vi "PicoScope2000ExampleBlock.vi"() -> ()   [LabVIEW 2017]
uses:
  PS2000.dll
panel:
  out "Handle in":i16
  out "handle out":i16
  in  "Sweeps":u32
  in  "Sweep Type":enum16{"Up", "Down", "Up/Down", "Down/Up"}(ring)
  in  "Dwell Time":sgl
  in  "Increment":sgl
  in  "Stop Frequency":sgl=1000.0
  in  "Start Frequency":sgl=1000.0
  in  "Waveform Type":T1(ring)
  in  "Peak to Peak":u32=1000000
  in  "Offset Voltage":i32
  in  "Source":i16(ring)=5 items=["Ch A", "Ch B", "Ch C", "Ch D", "Ext", "None"]
  in  "Voltage mV":i16=1400 min=0 max=20000 step=1
  out "Max number of samples you can use":i32=3967
  in  "Range":i16(ring)=8 items=["20V"=10, "10V"=9, "5V"=8, "2V"=7, "1V"=6, "500mV"=5, "200mV"=4, "100mV"=3, "50mV"=2]
  in  "Range":i16(ring)=8 items=["20V"=10, "10V"=9, "5V"=8, "2V"=7, "1V"=6, "500mV"=5, "200mV"=4, "100mV"=3, "50mV"=2]
  out "?":waveform(dbl)[](graph)=[{"t0"=timestamp(3612161019.70979 s since 1904-01-01), "dt"=8e-08, "Y"=array[1256 elements]}, {"t0"=timestamp(3612161019.70979 s since 1904-01-01), "dt"=8e-08, "Y"=array[1256 elements]}, {"t0"=timestamp(3612161019.70979 s since 1904-01-01), "dt"=8e-08, "Y"=array[1256 elements]}, {"t0"=timestamp(3612161019.70979 s since 1904-01-01), "dt"=8e-08, "Y"=array[1256 elements]}]
  in  "Enabled":bool=TRUE
  in  "Enabled":bool=TRUE
  in  "DC":i16(ring) items=["AC", "DC"]
  in  "DC":i16(ring)=1 items=["AC", "DC"]
  in  "No. of samples":i32=1256 min=0
  in  "Timebase":i16=3 min=0 max=14 step=1
  in  "Auto Trigger ms":i16 min=0 max=5000 step=100
  in  "Delay":i16 min=-100 max=100 step=1
  in  "Direction":i16(ring) items=["Rising", "Falling"]
  in  "stop":bool
  # "Trigger"
  # "Channel A"
  # "Channel B"
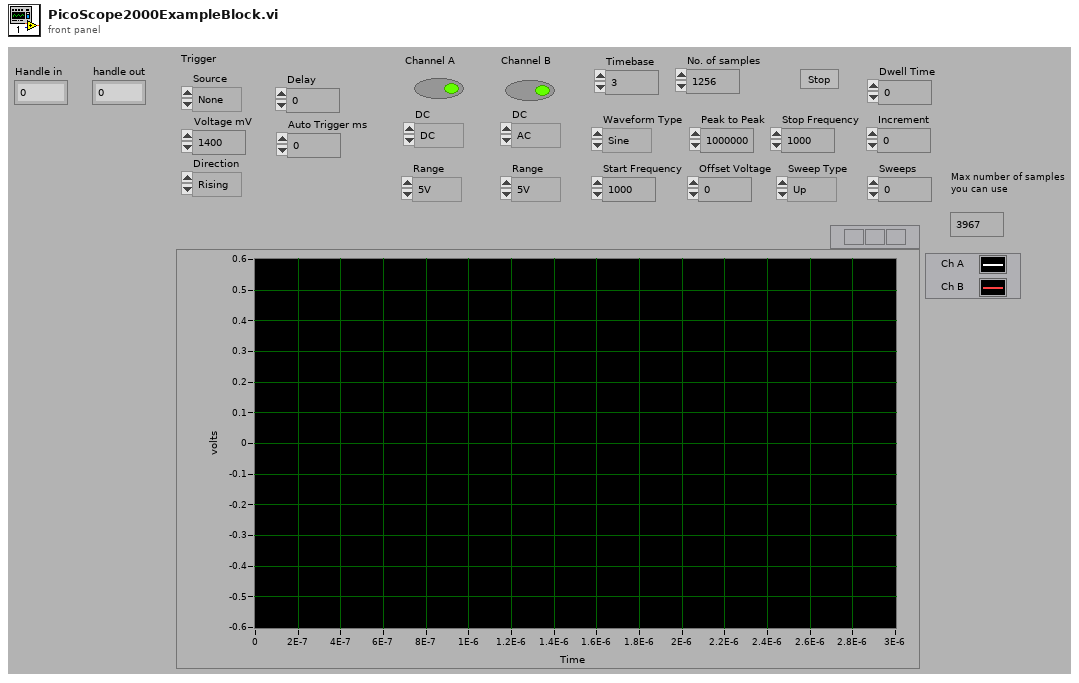
[diagram p1: front panel]
types:
  T1 = enum16{"Sine", "Square", "Triangle", "Rampup", "Rampdown"}
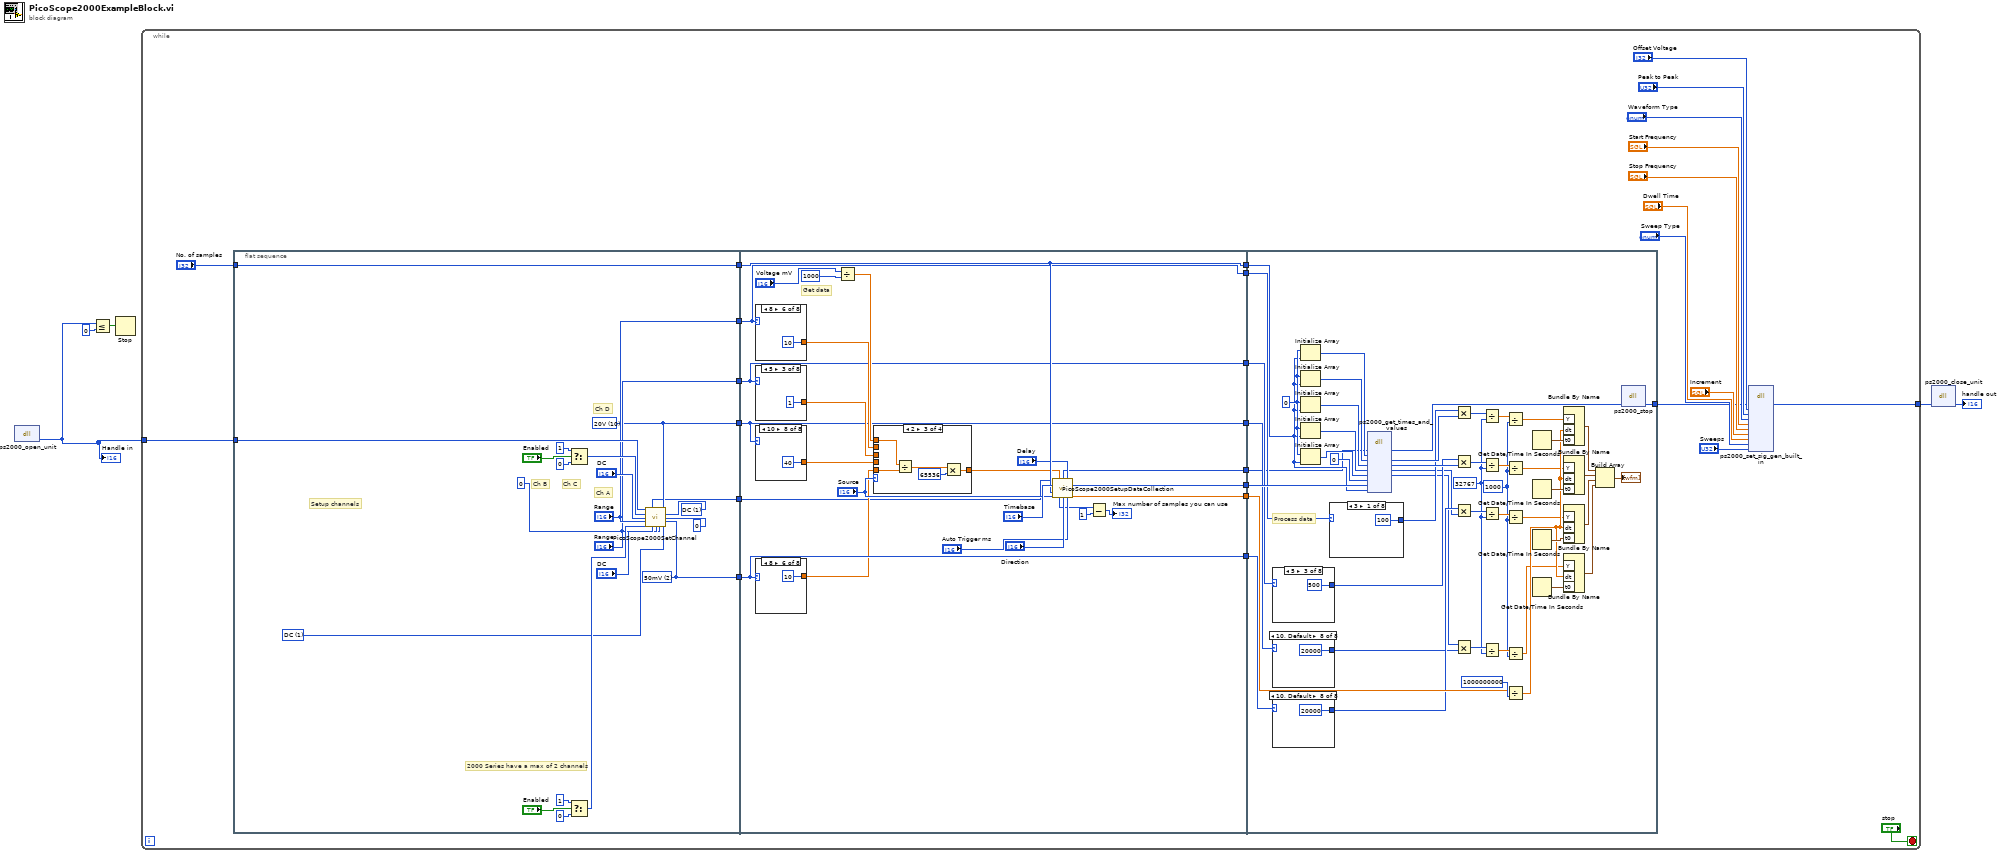
[diagram p0: block diagram]
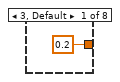
[diagram p2: hidden frame]
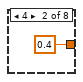
[diagram p3: hidden frame]
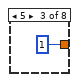
[diagram p4: hidden frame]
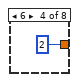
[diagram p5: hidden frame]
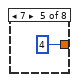
[diagram p6: hidden frame]
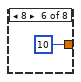
[diagram p7: hidden frame]
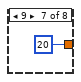
[diagram p8: hidden frame]
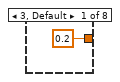
[diagram p9: hidden frame]
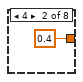
[diagram p10: hidden frame]
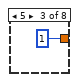
[diagram p11: hidden frame]
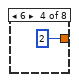
[diagram p12: hidden frame]
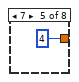
[diagram p13: hidden frame]
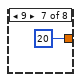
[diagram p14: hidden frame]
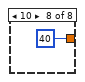
[diagram p15: hidden frame]
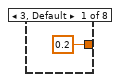
[diagram p16: hidden frame]
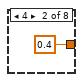
[diagram p17: hidden frame]
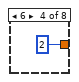
[diagram p18: hidden frame]
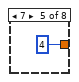
[diagram p19: hidden frame]
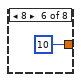
[diagram p20: hidden frame]
diagram:
  n1 = dll-call lib="PS2000.dll" fn="ps2000_open_unit" label="OpenUnit"() -> ("Handle"=w2:i16)  [unwired: 3 in, 2 out]
  "Handle in" <- w2
  n2 = Less Or Equal?(x=w2, y=i16 0) -> (x <= y?=w4:bool)
  n3 = Stop(stop? (T)=w4) -> ()
  n4 = while {
    tunnel: w2 -> [w32]
    tunnel: [w20] -> w5
    stop <- "stop" stop-if-true
    n5 = flat-sequence {
      tunnel: w32 -> [w48]
      tunnel: "No. of samples" -> [w34]
      tunnel: [w34] -> w19
      tunnel: [w35] -> w18
      tunnel: ["Range"] -> w17
      tunnel: ["Range"] -> w16
      tunnel: [w39] -> w15
      tunnel: [w38] -> w14
      tunnel: w19 -> [w75]
      tunnel: [w55] -> w13
      tunnel: w18 -> [w56]
      tunnel: [w75] -> w12
      tunnel: [w76] -> w11
      tunnel: w17 -> [w62]
      tunnel: [w62] -> w10
      tunnel: w16 -> [w63]
      tunnel: [w63] -> w9
      tunnel: [w74] -> w8
      tunnel: w15 -> [w60]
      tunnel: [w60] -> w7
      tunnel: w14 -> [w59]
      tunnel: [w59] -> w6
      tunnel: [w132] -> w21
      tunnel: w13 -> [w133]
      tunnel: w12 -> [w137]
      tunnel: w11 -> [w177]
      tunnel: w10 -> [w164]
      tunnel: w9 -> [w165]
      tunnel: w8 -> [w162]
      tunnel: w7 -> [w151]
      tunnel: w6 -> [w150]
      frame #0 {
        w40 = i16 1 items=["AC", "DC"] ("DC")
        w38 = i16 10 items=["20V"=10, "10V"=9, "5V"=8, "2V"=7, "1V"=6, "500mV"=5, "200mV"=4, "100mV"=3, "50mV"=2] ("Range")
        w41 = i16 1 items=["AC", "DC"] ("DC")
        w39 = i16 2 items=["20V"=10, "10V"=9, "5V"=8, "2V"=7, "1V"=6, "500mV"=5, "200mV"=4, "100mV"=3, "50mV"=2] ("Range")
        # "2000 Series have a max of 2 channels"
        # "Ch C"
        # "Ch D"
        # "Ch B"
        # "Ch A"
        # "Setup channels"
        n6 = Select(t=1, s="Enabled", f=0) -> (s? t:f=w47:i32)
        n7 = Select(t=1, s="Enabled", f=0) -> (s? t:f=w44:i32)
        n8 = call "PicoScope2000SetChannel.vi"("Handle in"=w48, "Channel D range"=w38, "Channel A enabled"=w47, "Channel D dc"=w40, "Channel A dc"="DC", "Channel D enabled"=0, "Channel A range"="Range", "Channel C range"=w39, "Channel B enabled"=w44, "Channel B dc"="DC", "Channel B range"="Range", "Channel C enabled"=0, "Channel C dc"=w41) -> ("Handle out"=w35:i16)  [unwired: 2 in]
      }
      frame #1 {
        # "Get data"
        n9 = case shown="8" w62 {
          tunnel: [0.2 0.4 1 2 4 10 20 40] -> w66
          frame 3, Default {
          }
          frame 4 {
          }
          frame 5 {
          }
          frame 6 {
          }
          frame 7 {
          }
          frame 8 {
          }
          frame 9 {
          }
          frame 10 {
          }
        }
        n10 = case shown="5" w63 {
          tunnel: [0.2 0.4 1 2 4 10 20 40] -> w65
          frame 3, Default {
          }
          frame 4 {
          }
          frame 5 {
          }
          frame 6 {
          }
          frame 7 {
          }
          frame 8 {
          }
          frame 9 {
          }
          frame 10 {
          }
        }
        n11 = case shown="10" w59 {
          tunnel: [0.2 0.4 1 2 4 10 20 40] -> w57
          frame 3, Default {
          }
          frame 4 {
          }
          frame 5 {
          }
          frame 6 {
          }
          frame 7 {
          }
          frame 8 {
          }
          frame 9 {
          }
          frame 10 {
          }
        }
        n12 = case shown="8" w60 {
          tunnel: [0.2 0.4 1 2 4 10 20 40] -> w58
          frame 3, Default {
          }
          frame 4 {
          }
          frame 5 {
          }
          frame 6 {
          }
          frame 7 {
          }
          frame 8 {
          }
          frame 9 {
          }
          frame 10 {
          }
        }
        n13 = Divide(x="Voltage mV", y=1000) -> (x/y=w67:dbl)
        n14 = case shown="2" "Source" {
          tunnel: w66 -> [w115 _ _ _]
          tunnel: w65 -> [_ w117 _ _]
          tunnel: w67 -> [w116 w118 w123 w128]
          tunnel: [w112 w119 w124 w129] -> w61
          tunnel: w58 -> [_ _ w122 _]
          tunnel: w57 -> [_ _ _ w127]
          frame 0, Default {
            n15 = Divide(x=w116, y=w115) -> (x/y=w114:dbl)
            n16 = Multiply(x=w114, y=65536) -> (x*y=w112:dbl)
          }
          frame 1 {
            n17 = Divide(x=w118, y=w117) -> (x/y=w121:dbl)
            n18 = Multiply(x=w121, y=65536) -> (x*y=w119:dbl)
          }
          frame 2 {
            n19 = Divide(x=w123, y=w122) -> (x/y=w126:dbl)
            n20 = Multiply(x=w126, y=65536) -> (x*y=w124:dbl)
          }
          frame 3 {
            n21 = Divide(x=w128, y=w127) -> (x/y=w131:dbl)
            n22 = Multiply(x=w131, y=65536) -> (x*y=w129:dbl)
          }
        }
        n23 = call "PicoScope2000SetupDataCollection.vi"("Handle in"=w56, "Threshold"=w61, "Delay"="Delay", "Timebase"="Timebase", "No of samples"=w75, "Source"="Source", "Direction"="Direction", "Auto Trigger ms"="Auto Trigger ms") -> ("Handle out"=w55:i16, "time units"=w76:i16, "Max Samples"=w71:i32, "time_interval_ns"=w74:dbl)  [unwired: 2 in, 2 out]
        n24 = Subtract(x=w71, y=1) -> (x-y=→"Max number of samples you can use":i32)
      }
      frame #2 {
        w154 = 1000
        w155 = 32767
        w138 = 0
        # "Process data"
        n25 = case shown="5" w165 {
          tunnel: [100 200 500 1000 2000 5000 10000 20000] -> w167
          frame 3 {
          }
          frame 4 {
          }
          frame 5 {
          }
          frame 6 {
          }
          frame 7 {
          }
          frame 8 {
          }
          frame 9 {
          }
          frame 10, Default {
          }
        }
        n26 = case shown="10, Default" w150 {
          tunnel: [100 200 500 1000 2000 5000 10000 20000] -> w156
          frame 3 {
          }
          frame 4 {
          }
          frame 5 {
          }
          frame 6 {
          }
          frame 7 {
          }
          frame 8 {
          }
          frame 9 {
          }
          frame 10, Default {
          }
        }
        n27 = case shown="10, Default" w151 {
          tunnel: [100 200 500 1000 2000 5000 10000 20000] -> w157
          frame 3 {
          }
          frame 4 {
          }
          frame 5 {
          }
          frame 6 {
          }
          frame 7 {
          }
          frame 8 {
          }
          frame 9 {
          }
          frame 10, Default {
          }
        }
        n28 = Initialize Array(w138, w137) -> (w135:i32[])
        n29 = Initialize Array(w138, w137) -> (w181:i32[])
        n30 = Initialize Array(w138, w137) -> (w180:i32[])
        n31 = Initialize Array(w138, w137) -> (w179:i32[])
        n32 = Initialize Array(w138, w137) -> (w178:i32[])
        n33 = case shown="3" w164 {
          tunnel: [100 200 500 1000 2000 5000 10000 20000] -> w166
          frame 3 {
          }
          frame 4 {
          }
          frame 5 {
          }
          frame 6 {
          }
          frame 7 {
          }
          frame 8 {
          }
          frame 9 {
          }
          frame 10, Default {
          }
        }
        n34 = dll-call lib="PS2000.dll" fn="ps2000_get_times_and_values" label="GetTimes&Values"("handle"=w133, "times"=w135, "bufferA"=w181, "bufferB"=w180, "bufferC"=w179, "bufferD"=w178, "overflow"=0, "times_units"=w177, "numValues"=w137) -> ("handle"=w173:i16, "bufferA"=w174:i16[], "bufferB"=w168:i16[], "bufferC"=w153:i16[], "bufferD"=w152:i16[])  [unwired: 8 in, 2 out]
        n35 = Multiply(x=w166, y=w174) -> (x*y=w176:i32[])
        n36 = Multiply(x=w167, y=w168) -> (x*y=w171:i32[])
        n37 = Multiply(x=w157, y=w153) -> (x*y=w161:i32[])
        n38 = Multiply(x=w152, y=w156) -> (x*y=w159:i32[])
        n39 = Divide(x=w176, y=w155) -> (x/y=w175:dbl[])
        n40 = Divide(x=w171, y=w155) -> (x/y=w170:dbl[])
        n41 = Divide(x=w161, y=w155) -> (x/y=w160:dbl[])
        n42 = Divide(x=w159, y=w155) -> (x/y=w158:dbl[])
        n43 = Divide(x=w175, y=w154) -> (x/y=w141:dbl[])
        n44 = Divide(x=w170, y=w154) -> (x/y=w134:dbl[])
        n45 = Divide(x=w160, y=w154) -> (x/y=w140:dbl[])
        n46 = Divide(x=w158, y=w154) -> (x/y=w139:dbl[])
        n47 = Divide(x=w162, y=1000000000) -> (x/y=w147:dbl)
        n48 = Get Date/Time In Seconds() -> (seconds since 1Jan1904=w172:timestamp)
        n49 = Get Date/Time In Seconds() -> (seconds since 1Jan1904=w169:timestamp)
        n50 = Get Date/Time In Seconds() -> (seconds since 1Jan1904=w149:timestamp)
        n51 = Get Date/Time In Seconds() -> (seconds since 1Jan1904=w148:timestamp)
        n52 = Bundle By Name("Y"=w141, "dt"=w147, "t0"=w172) -> (w146:waveform(dbl))  [unwired: 1 in]
        n53 = Bundle By Name("Y"=w134, "dt"=w147, "t0"=w169) -> (w143:waveform(dbl))  [unwired: 1 in]
        n54 = Bundle By Name("Y"=w140, "dt"=w147, "t0"=w149) -> (w144:waveform(dbl))  [unwired: 1 in]
        n55 = Bundle By Name("Y"=w139, "dt"=w147, "t0"=w148) -> (w145:waveform(dbl))  [unwired: 1 in]
        n56 = Build Array(w146, w143, w144, w145) -> (→"?":waveform(dbl)[])
        n57 = dll-call lib="PS2000.dll" fn="ps2000_stop" label="Stop"("handle"=w173) -> ("handle"=w132:i16)  [unwired: 4 in, 2 out]
      }
    }
    n58 = dll-call lib="PS2000.dll" fn="ps2000_set_sig_gen_built_in"("handle"=w21, "offsetvoltage"="Offset Voltage", "pktopk"="Peak to Peak", "wavetype"="Waveform Type", "startfrequency"="Start Frequency", "stopfrequency"="Stop Frequency", "increment"="Increment", "dwelltime"="Dwell Time", "sweeptype"="Sweep Type", "sweeps"="Sweeps") -> ("handle"=w20:i16)  [unwired: 13 in, 2 out]
  }
  n59 = dll-call lib="PS2000.dll" fn="ps2000_close_unit" ("ps3000.dll:_ps3000_close_unit@4")("handle"=w5) -> ("handle"=→"handle out":i16)  [unwired: 4 in, 2 out]
